vi "DAQ comm.vi"(7 "DAQ T state cluster in":T1={"DAQ state"=enum."Global comm", "device"="Dev1", "start (ms)"=0, "error"={"status"=FALSE, "code"=0, "source"=""}, "T cont"={"exec"={"T mode"=enum."Setting up", "log"=FALSE, "thermistor"=enum."solo"}, "T status"={"Temp"=0.0}, "utility"={"meas index"=300, "wait (ms)"=0, "therm volt"=0.0, "t T hist"=[]}}} {"T cont"."utility"."therm volt" format="%_6g"; "T cont"."T status"."Temp" format="%_6g"}) -> (8 "DAQ T state cluster out":T1={"DAQ state"=enum."Global comm", "device"="Dev1", "start (ms)"=0, "error"={"status"=FALSE, "code"=0, "source"=""}, "T cont"={"exec"={"T mode"=enum."Listening to exec", "log"=FALSE, "thermistor"=enum."solo"}, "T status"={"Temp"=0.0}, "utility"={"meas index"=0, "wait (ms)"=0, "therm volt"=0.0, "t T hist"=[]}}} {"T cont"."utility"."therm volt" format="%_6g"; "T cont"."T status"."Temp" format="%_6g"})   [LabVIEW 2019]
doc: "This subVI is one of the states of the DAQ state machine in the thermistor experiment.\n\nThis state monitors the global variables used in the thermistor experiment. Depending upon the T control mode, it can be transient, or a dwell state with indefinite dwell time while waiting to engage the DAQ interfacing.\n\nPaul K Dixon\nP3600\nCSUSB Physics"
uses:
  typedefs/DAQ T state cluster.ctl
  typedefs/DAQ T state enum.ctl
  typedefs/temp cont cluster.ctl
  typedefs/temp exec cluster.ctl
  typedefs/temp mode enum.ctl
  typedefs/temp indicator.ctl
  typedefs/temp cont utility.ctl
  globals/Bug man temp globals.vi
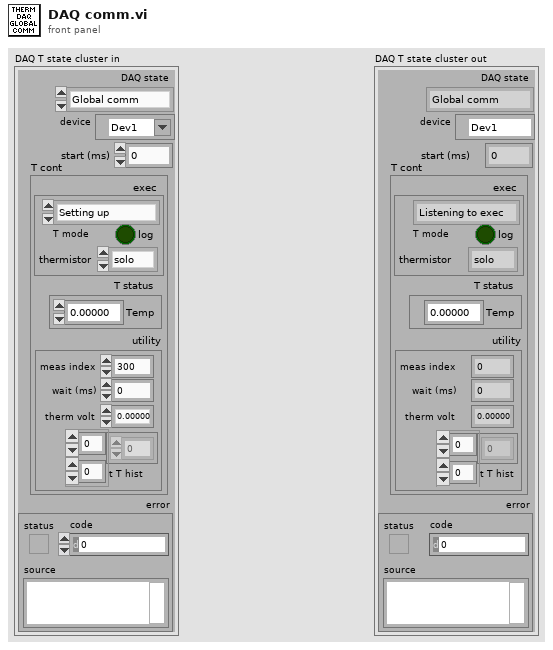
[diagram p1: front panel]
types:
  T1 = typedef "DAQ T state cluster.ctl" = cluster{"DAQ state":T2, "device":tag, "start (ms)":i32, "error":errorcluster, "T cont":T3}
  T2 = typedef "DAQ T state enum.ctl" = enum16{"Global comm", "Meas T ", "Wait", "Exit"}
  T3 = typedef "temp cont cluster.ctl" = cluster{"exec":T4, "T status":T6, "utility":T7}
  T4 = typedef "temp exec cluster.ctl" = cluster{"T mode":T5, "log":bool, "thermistor":enum16{"solo", "bug"}}
  T5 = typedef "temp mode enum.ctl" = enum16{"Setting up", "Listening to exec", "Exit"}
  T6 = typedef "temp indicator.ctl" = cluster{"Temp":dbl}
  T7 = typedef "temp cont utility.ctl" = cluster{"meas index":i32, "wait (ms)":i32, "therm volt":dbl, "t T hist":dbl[][]}
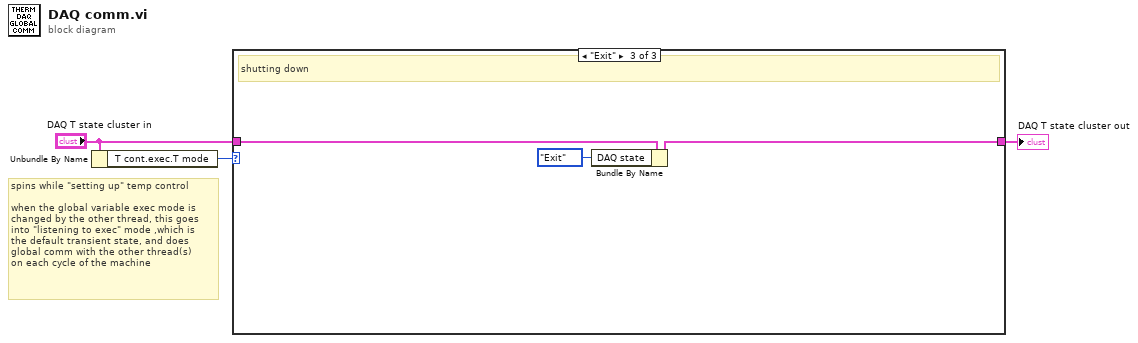
[diagram p0: block diagram]
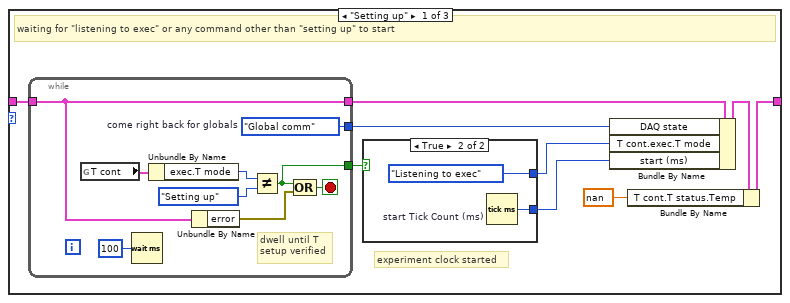
[diagram p2: hidden frame]
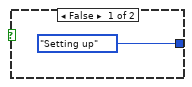
[diagram p3: hidden frame]
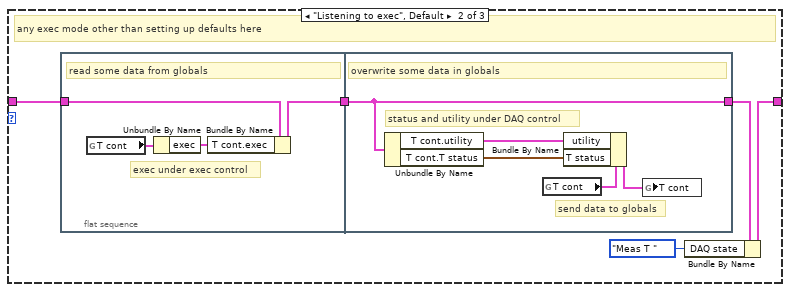
[diagram p4: hidden frame]
diagram:
  # "spins while \"setting up\" temp control \n\nwhen the global variable exec mode is\nchanged by the other thread, this goes \ninto \"listening to exec\" mode ,which is\nthe default transient state, and does \nglobal comm with the other thread(s)\non each cycle of the machine"
  n1 = Unbundle By Name("DAQ T state cluster in") -> ("T cont.exec.T mode"=w3:T5)
  n2 = case shown="\"Exit\"" w3 {
    tunnel: "DAQ T state cluster in" -> [w12 w29 w41]
    tunnel: [w5 w28 w40] -> w1
    frame "Setting up" {
      # "experiment clock started"
      # "waiting for \"listening to exec\" or any command other than \"setting up\" to start"
      n3 = while {
        tunnel: w12 -> [w22]
        tunnel: [w22] -> w11
        tunnel: [w20] -> w10
        tunnel: [w16] -> w8
        stop <- w24 stop-if-true
        w20 = DAQ_T_state_enum."Global comm"  # come right back for globals
        # "dwell until T \nsetup verified"
        n4 = global read "Bug man temp globals.vi" "T cont"() -> (w19:T3)
        n5 = Wait (ms)(milliseconds to wait=u32 100) -> ()  [unwired: 1 out]
        n6 = Unbundle By Name(w19) -> ("exec.T mode"=w18:T5)
        n7 = Unbundle By Name(w22) -> ("error"=w23:errorcluster)
        n8 = Not Equal?(x=w18, y=temp_mode_enum."Setting up" ("exec.T mode")) -> (x != y?=w16:bool)
        n9 = Compound Arithmetic op=OR(w16, w23) -> (w24:bool)
      }
      n10 = case shown="True" w8 {
        tunnel: [temp_mode_enum."Setting up" ("T cont.exec.T mode") temp_mode_enum."Listening to exec" ("T cont.exec.T mode")] -> w9
        tunnel: [_ w14] -> w7
        frame False {
        }
        frame True {
          n11 = Tick Count (ms) "start Tick Count (ms)"() -> (millisecond timer value=w14:u32)
        }
      }
      n12 = Bundle By Name(cluster=w11, "DAQ state"=w10, "T cont.exec.T mode"=w9, "start (ms)"=w7) -> (w6:T1)
      n13 = Bundle By Name(cluster=w6, "T cont.T status.Temp"=nan) -> (w5:T1)
    }
    frame "Listening to exec", Default {
      # "any exec mode other than setting up defaults here"
      n14 = flat-sequence {
        tunnel: w29 -> [w33]
        tunnel: [w30] -> w26
        tunnel: [w34] -> w27
        tunnel: w26 -> [w34]
        frame #0 {
          # "exec under exec control"
          # "read some data from globals"
          n15 = global read "Bug man temp globals.vi" "T cont"() -> (w32:T3)
          n16 = Unbundle By Name(w32) -> ("exec"=w31:T4)
          n17 = Bundle By Name(cluster=w33, "T cont.exec"=w31) -> (w30:T1)
        }
        frame #1 {
          # "status and utility under DAQ control"
          # "send data to globals"
          # "overwrite some data in globals"
          n18 = Unbundle By Name(w34) -> ("T cont.utility"=w35:T7, "T cont.T status"=w36:T6)
          n19 = global read "Bug man temp globals.vi" "T cont"() -> (w38:T3)
          n20 = Bundle By Name(cluster=w38, "utility"=w35, "T status"=w36) -> (w37:T3)
          n21 = global write "Bug man temp globals.vi" "T cont"(w37) -> ()
        }
      }
      n22 = Bundle By Name(cluster=w27, "DAQ state"=DAQ_T_state_enum."Meas T ") -> (w28:T1)
    }
    frame "Exit" {
      # "shutting down"
      n23 = Bundle By Name(cluster=w41, "DAQ state"=DAQ_T_state_enum."Exit") -> (w40:T1)
    }
  }
  "DAQ T state cluster out" <- w1
